vi "Measure Clock Frequency.vi"() -> (3 "Measured Clock Frequence [Hz]":dbl)   [LabVIEW 2021]
uses:
  <vilib>/ptbypt/NI_PtbyPt.lvlib
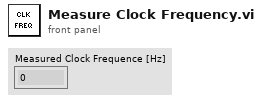
[diagram p1: front panel]
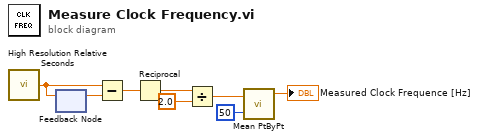
[diagram p0: block diagram]
diagram:
  n1 = call <vilib>:"High Resolution Relative Seconds.vi"() -> ("relative seconds"=w1:dbl)
  n2 = feedback #1() -> (w2:dbl)  [unwired: 1 in]
  n3 = feedback-in #1(w1) -> ()
  n4 = Subtract(x=w1, y=w2) -> (x-y=w3:dbl)
  n5 = Reciprocal(x=w3) -> (1/x=w4:dbl)
  n6 = Divide(x=w4, y=2.0) -> (x/y=w6:dbl)
  n7 = call <vilib>:"Mean PtByPt.vi"("x"=w6, "sample length"=50) -> ("mean"=→"Measured Clock Frequence [Hz]":dbl)  [unwired: 2 in, 1 out]
